vi "Set PID.vi"(8 "error in (no error)":errorcluster, 10 "Control Parameters":cluster{"P":dbl, "I":dbl, "D":u16}, 11 "Lakeshore 325 in":refnum<class "Lakeshore 325.lvclass">) -> (0 "error out":errorcluster, 3 "Lakeshore 325 out":refnum<class "Lakeshore 325.lvclass">)   [LabVIEW 2022 SP3, in "Lakeshore 325.lvclass"]
uses:
  Lakeshore 325.lvclass
  Lakeshore 325.lvclass/Lakeshore 325.ctl
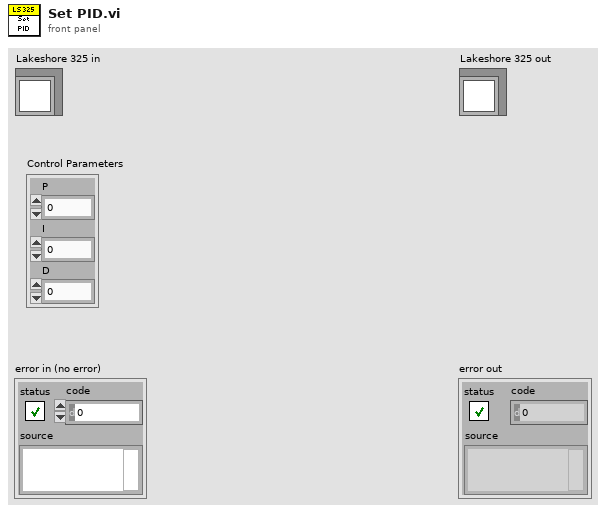
[diagram p1: front panel]
types:
  T1 = typedef "Lakeshore 325.lvclass/Lakeshore 325 Temp Control Parameters.ctl" = cluster{"Mode":u16, "Setpoint":dbl, "Manual Power (%)":dbl, "Control Parameters":cluster{"P":dbl, "I":dbl, "D":u16}}
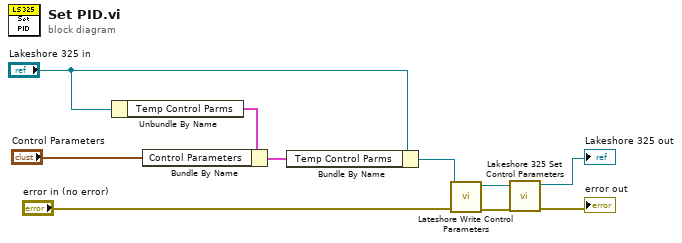
[diagram p0: block diagram]
diagram:
  n1 = Unbundle By Name("Lakeshore 325 in") -> ("Temp Control Parms"=w10:T1)
  n2 = Bundle By Name(cluster=w10, "Control Parameters"="Control Parameters") -> (w7:T1)
  n3 = Bundle By Name(cluster="Lakeshore 325 in", "Temp Control Parms"=w7) -> (w4:refnum<class "Lakeshore 325.lvclass">)
  n4 = call "Lateshore Write Control Parameters.vi"("error in (no error)"="error in (no error)", "Lakeshore 325 in"=w4) -> ("error out"=w1:errorcluster, "Lakeshore 325 out"=w2:refnum<class "Lakeshore 325.lvclass">)  [unwired: 8 in]
  n5 = call "Lakeshore 325 Set Control Parameters.vi"("error in (no error)"=w1, "Lakeshore 325 in"=w2) -> ("error out"=→"error out":errorcluster, "Lakeshore 325 out"=→"Lakeshore 325 out":refnum<class "Lakeshore 325.lvclass">)  [unwired: 8 in]
